vi "Trapezoidal Acceleration.vi"(6 "Skip":dbl, 8 "AccelRate":dbl, 9 "Desired":dbl, 10 "Actual":dbl, 11 "LoopTime":dbl) -> (2 "New Actual":dbl)   [LabVIEW 2013]
doc: "Fixes motor acceleration to a linear rate."
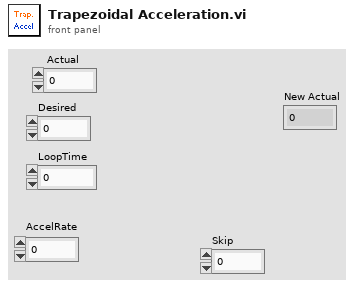
[diagram p1: front panel]
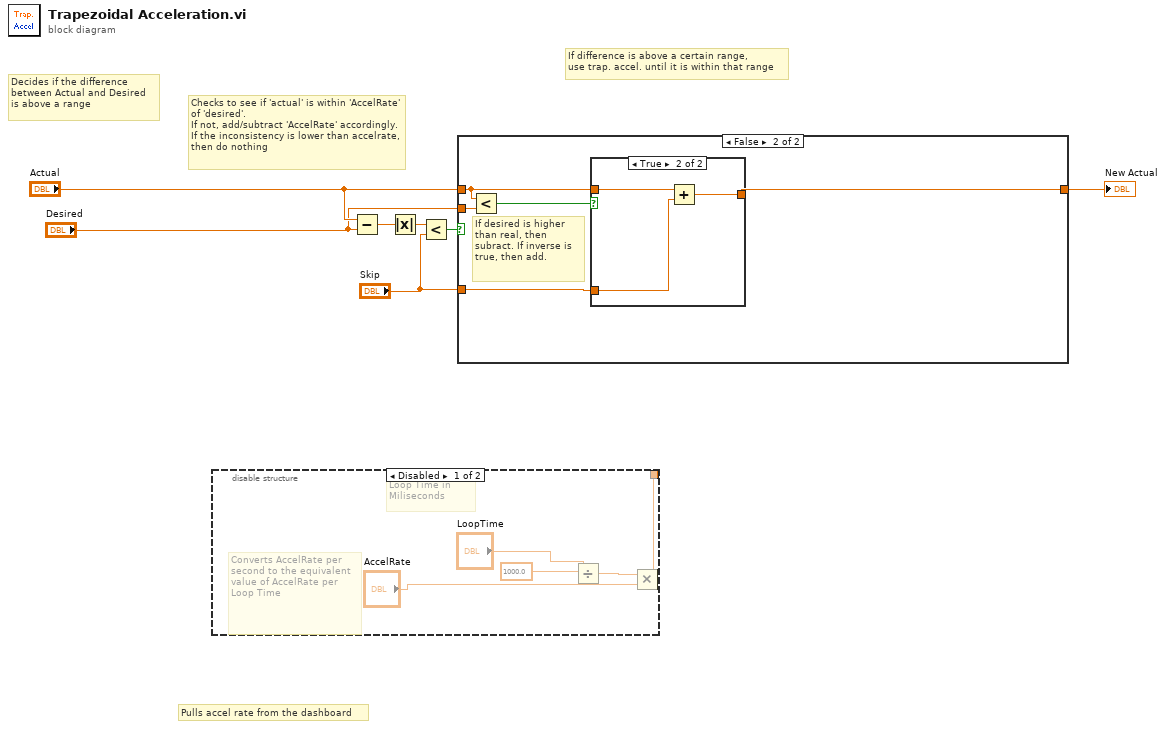
[diagram p0: block diagram]
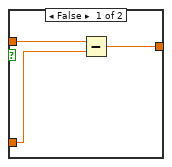
[diagram p4: hidden frame]
diagram:
  # "If difference is above a certain range,\nuse trap. accel. until it is within that range"
  # "Pulls accel rate from the dashboard"
  # "Checks to see if 'actual' is within 'AccelRate' of 'desired'.\nIf not, add/subtract 'AccelRate' accordingly. If the inconsistency is lower than accelrate, then do nothing"
  # "Decides if the difference\nbetween Actual and Desired\nis above a range"
  n1 = disable-structure shown="Disabled" {
    disable-tunnel: [w10 _] -> _
    frame Disabled {
      # "Converts AccelRate per second to the equivalent value of AccelRate per Loop Time"
      # "Loop Time in Miliseconds"
      n2 = Divide(x="LoopTime", y=1000.0) -> (x/y=w11:dbl)
      n3 = Multiply(x=w11, y="AccelRate") -> (x*y=w10:dbl)
    }
    frame Enabled {
    }
  }
  n4 = Subtract(x="Actual", y="Desired") -> (x-y=w3:dbl)
  n5 = Absolute Value(x=w3) -> (abs(x)=w4:dbl)
  n6 = Less?(x=w4, y="Skip") -> (x < y?=w2:bool)
  n7 = case shown="False" w2 {
    tunnel: [w13 w18] -> w7
    tunnel: "Actual" -> [_ w17]
    tunnel: "Desired" -> [w13 w15]
    tunnel: "Skip" -> [_ w14]
    frame True {
    }
    frame False {
      # "If desired is higher than real, then subract. If inverse is true, then add."
      n8 = Less?(x=w17, y=w15) -> (x < y?=w16:bool)
      n9 = case shown="True" w16 {
        tunnel: w17 -> [w20 w23]
        tunnel: [w21 w24] -> w18
        tunnel: w14 -> [w19 w22]
        frame False {
          n10 = Subtract(x=w20, y=w19) -> (x-y=w21:dbl)
        }
        frame True {
          n11 = Add(x=w23, y=w22) -> (x+y=w24:dbl)
        }
      }
    }
  }
  "New Actual" <- w7
